vi "Oven_Logs.vi"(6 "Oven Staion NAME":string, 7 "SQl IN":T1, 8 "Oven Data":u16[](array[numeric]), 9 "Oven Staion ID":string, 10 "Shift":i32, 11 "PLC Data":T3[](array[typedef])) -> (3 "output cluster":T2)   [LabVIEW 2017]
doc: "This vi is used to create logs for OVEN -- all oven signasls are taken from delta oven plc and 4 pressure and time signals are taken from press.. CID of press and CID/ID of oven number is used to sync both signals."
uses:
  Control/Main_Data.ctl
  <vilib>/addons/database/Connection.llb/Conn ObjectReference.ctl
  <vilib>/addons/database/NI_Database_API.lvlib
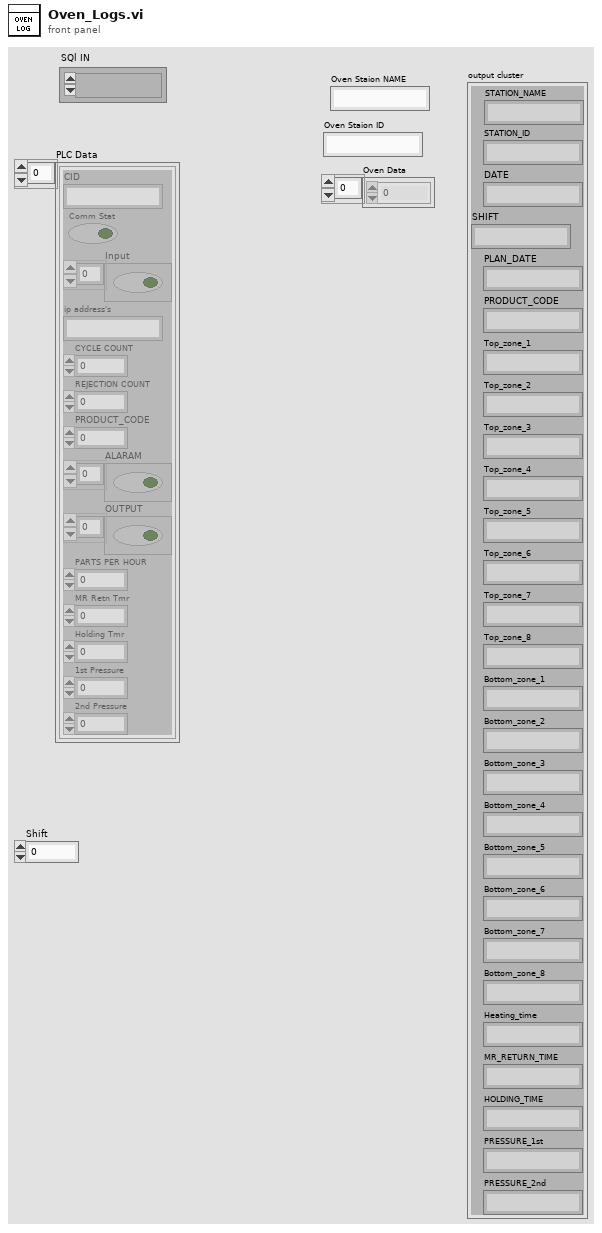
[diagram p1: front panel]
types:
  T1 = typedef "NI_Database_API.lvlib/Conn ObjectReference.ctl" = refnum<k1>
  T2 = cluster{"STATION_ID":string, "DATE":string, "SHIFT":string, "PLAN_DATE":string, "PRODUCT_CODE":string, "Top_zone_1":string, "Top_zone_2":string, "Top_zone_3":string, "Top_zone_4":string, "Top_zone_5":string, "Top_zone_6":string, "Top_zone_7":string, "Top_zone_8":string, "Bottom_zone_1":string, "Bottom_zone_2":string, "Bottom_zone_3":string, "Bottom_zone_4":string, "Bottom_zone_5":string, "Bottom_zone_6":string, "Bottom_zone_7":string, "Bottom_zone_8":string, "Heating_time":string, "MR_RETURN_TIME":string, "HOLDING_TIME":string, "PRESSURE_1st":string, "PRESSURE_2nd":string, "STATION_NAME":string}
  T3 = typedef "Main_Data.ctl" = cluster{"CID":string, "Comm Stat":bool, "Input":bool[], "ip address's":string, "CYCLE COUNT":u32, "REJECTION COUNT":u32, "PRODUCT_CODE":i16, "ALARAM":bool[], "OUTPUT":bool[], "PARTS PER HOUR":i16, "MR Retn Tmr":dbl, "Holding Tmr":dbl, "1st Pressure":dbl, "2nd Pressure":dbl}
  T4 = typedef "LVDateTimeRec.ctl" = cluster{"fractional second":dbl, "second":i32, "minute":i32, "hour":i32, "day of month":i32, "month":i32, "year":i32, "day of week":i32, "day of year":i32, "DST":i32}
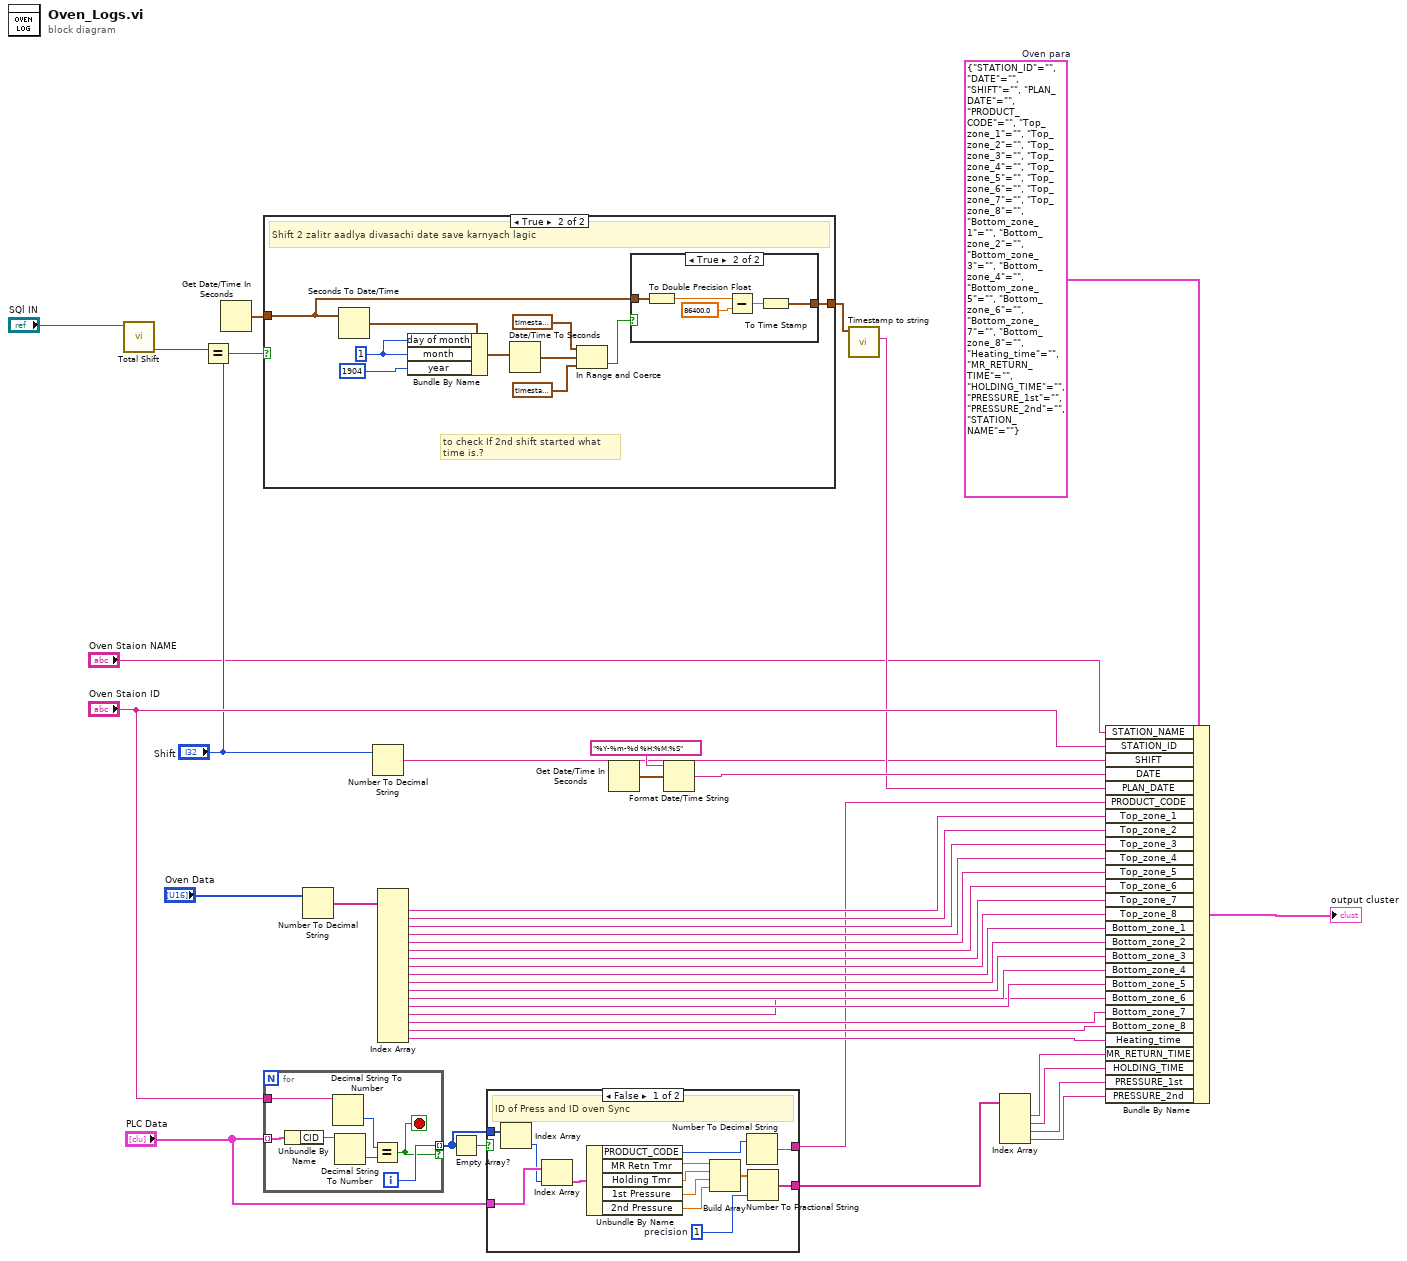
[diagram p0: block diagram]
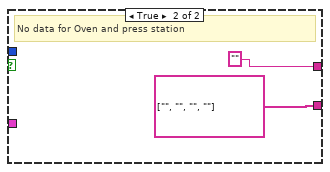
[diagram p4: hidden frame]
diagram:
  w42 = T2 {"STATION_ID"="", "DATE"="", "SHIFT"="", "PLAN_DATE"="", "PRODUCT_CODE"="", "Top_zone_1"="", "Top_zone_2"="", "Top_zone_3"="", "Top_zone_4"="", "Top_zone_5"="", "Top_zone_6"="", "Top_zone_7"="", "Top_zone_8"="", "Bottom_zone_1"="", "Bottom_zone_2"="", "Bottom_zone_3"="", "Bottom_zone_4"="", "Bottom_zone_5"="", "Bottom_zone_6"="", "Bottom_zone_7"="", "Bottom_zone_8"="", "Heating_time"="", "MR_RETURN_TIME"="", "HOLDING_TIME"="", "PRESSURE_1st"="", "PRESSURE_2nd"="", "STATION_NAME"=""}  # Oven para
  n1 = call "Total Shift.vi"("connection reference"="SQl IN") -> ("Total Shifts"=w10:i32)  [unwired: 9 in, 1 out]
  n2 = Equal?(x=w10, y="Shift") -> (x = y?=w9:bool)
  n3 = Get Date/Time In Seconds() -> (seconds since 1Jan1904=w8:timestamp)
  n4 = case shown="True" w9 {
    tunnel: w8 -> [w44 w45]
    tunnel: [w44 w46] -> w7
    frame False {
    }
    frame True {
      w51 = 1 ("day of month")
      # "to check If 2nd shift started what time is.?"
      # "Shift 2 zalitr aadlya divasachi date save karnyach lagic"
      n5 = Seconds To Date/Time(time stamp (now)=w45) -> (date time rec=w52:T4)  [unwired: 1 in]
      n6 = Bundle By Name(cluster=w52, "day of month"=w51, "month"=w51, "year"=1904) -> (w54:T4)
      n7 = Date/Time To Seconds(2:w54) -> (0:w50:timestamp)  [unwired: 1 in]
      n8 = In Range and Coerce(upper limit=timestamp(5399 s since 1904-01-01), x=w50, lower limit=timestamp(-19800 s since 1904-01-01)) -> (In Range?=w47:bool)  [unwired: 1 out]
      n9 = case shown="True" w47 {
        tunnel: [w55 w57] -> w46
        tunnel: w45 -> [w55 w56]
        frame False {
        }
        frame True {
          n10 = To Double Precision Float(number=w56) -> (double precision float=w60:dbl)
          n11 = Subtract(x=w60, y=86400.0) -> (x-y=w58:dbl)
          n12 = To Time Stamp(1:w58) -> (0:w57:timestamp)
        }
      }
    }
  }
  n13 = for {
    tunnel: "PLC Data" -> [w67] mode=indexing
    tunnel: "Oven Staion ID" -> [w65]
    tunnel: [w62] -> w40 mode=indexing if=w61
    i -> [w62]
    stop <- w61 stop-if-true
    n14 = Unbundle By Name(w67) -> ("CID"=w66:string)
    n15 = Decimal String To Number(string=w65) -> (number=w63:i32)  [unwired: 2 in, 1 out]
    n16 = Decimal String To Number(string=w66) -> (number=w64:i32)  [unwired: 2 in, 1 out]
    n17 = Equal?(x=w63, y=w64) -> (x = y?=w61:bool)
  }
  n18 = Number To Decimal String(number="Oven Data") -> (decimal integer string=w32:string[])  [unwired: 1 in]
  n19 = Number To Decimal String(number="Shift") -> (decimal integer string=w2:string)  [unwired: 1 in]
  n20 = Index Array(array=w32) -> (element #1=w31:string, element #2=w30:string, element #3=w29:string, element #4=w28:string, element #5=w27:string, element #6=w26:string, element #7=w25:string, element #8=w24:string, element #9=w23:string, element #10=w22:string, element #11=w21:string, element #12=w20:string, element #13=w19:string, element #14=w18:string, element #15=w17:string, element #16=w16:string, element #17=w15:string)  [unwired: 17 in]
  n21 = Empty Array?(array=w40) -> (empty?=w43:bool)
  n22 = case shown="False" w43 {
    tunnel: [w70 string[] ["", "", "", ""]] -> w39
    tunnel: "PLC Data" -> [w80 _]
    tunnel: w40 -> [w79 _]
    tunnel: [w68 "" ("2nd Pressure")] -> w14
    frame False {
      w75 = i16 1  # precision
      # "ID of Press and ID oven Sync"
      n23 = Index Array(array=w79) -> (element=w78:i32)  [unwired: 1 in]
      n24 = Index Array(array=w80, index=w78) -> (element=w77:T3)
      n25 = Unbundle By Name(w77) -> ("PRODUCT_CODE"=w69:i16, "MR Retn Tmr"=w74:dbl, "Holding Tmr"=w73:dbl, "1st Pressure"=w72:dbl, "2nd Pressure"=w71:dbl)
      n26 = Build Array(w74, w73, w72, w71) -> (w76:dbl[])
      n27 = Number To Decimal String(number=w69) -> (decimal integer string=w68:string)  [unwired: 1 in]
      n28 = Number To Fractional String(number=w76, precision (6)=w75) -> (F-format string=w70:string[])  [unwired: 2 in]
    }
    frame True {
      # "No data for Oven and press station"
    }
  }
  n29 = Get Date/Time In Seconds() -> (seconds since 1Jan1904=w12:timestamp)
  n30 = Format Date/Time String(time format string (%c)="%Y-%m-%d %H:%M:%S", seconds (now)=w12) -> (date/time string=w11:string)  [unwired: 1 in]
  n31 = call "Timestamp to string.vi"("time stamp"=w7) -> ("Date String"=w6:string)  [unwired: 8 in, 2 out]
  n32 = Index Array(array=w39) -> (element #1=w34:string, element #2=w35:string, element #3=w36:string, element #4=w37:string)  [unwired: 4 in]
  n33 = Bundle By Name(cluster=w42, "STATION_NAME"="Oven Staion NAME", "STATION_ID"="Oven Staion ID", "SHIFT"=w2, "DATE"=w11, "PLAN_DATE"=w6, "PRODUCT_CODE"=w14, "Top_zone_1"=w31, "Top_zone_2"=w30, "Top_zone_3"=w29, "Top_zone_4"=w28, "Top_zone_5"=w27, "Top_zone_6"=w26, "Top_zone_7"=w25, "Top_zone_8"=w24, "Bottom_zone_1"=w23, "Bottom_zone_2"=w22, "Bottom_zone_3"=w21, "Bottom_zone_4"=w20, "Bottom_zone_5"=w19, "Bottom_zone_6"=w18, "Bottom_zone_7"=w17, "Bottom_zone_8"=w16, "Heating_time"=w15, "MR_RETURN_TIME"=w34, "HOLDING_TIME"=w35, "PRESSURE_1st"=w36, "PRESSURE_2nd"=w37) -> (→"output cluster":T2)
